vi "Decision2(SubVI).vi"(0 "L_ind0":i32, 1 "number of sample":i32, 2 "L_ind1":i32, 3 "Peak_ind0":dbl[](array[numeric]), 4 "index":i32, 5 "Peak_ind1":dbl[](array[numeric])) -> (6 "L_sum":i32, 7 "Bits":dbl[](array[numeric]), 8 "Position":dbl[](array[numeric]))   [LabVIEW 2017]
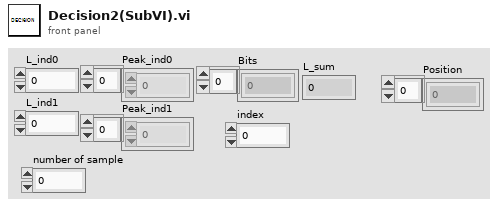
[diagram p1: front panel]
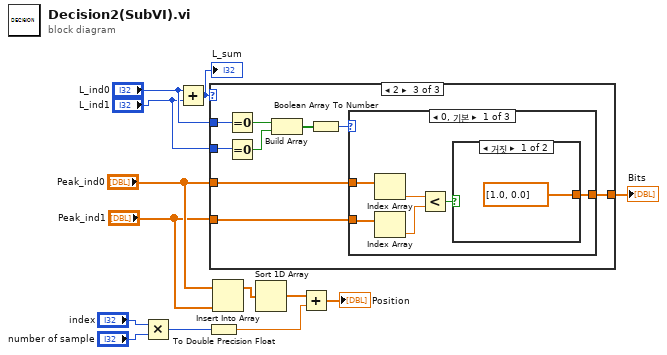
[diagram p0: block diagram]
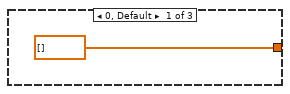
[diagram p2: hidden frame]
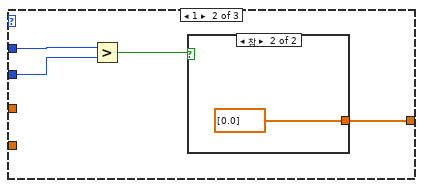
[diagram p3: hidden frame]
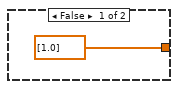
[diagram p4: hidden frame]
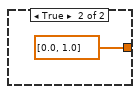
[diagram p5: hidden frame]
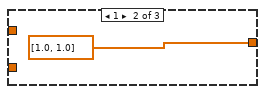
[diagram p6: hidden frame]
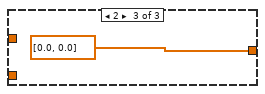
[diagram p7: hidden frame]
diagram:
  n1 = Multiply(x="index", y="number of sample") -> (x*y=w1:i32)
  n2 = Add(x="L_ind0", y="L_ind1") -> (x+y=w10:i32)
  "L_sum" <- w10
  n3 = To Double Precision Float(number=w1) -> (double precision float=w5:dbl)
  n4 = case shown="2" w10 {
    tunnel: [dbl[] [] w17 w23] -> w11
    tunnel: "L_ind0" -> [_ w16 w29]
    tunnel: "L_ind1" -> [_ w15 w28]
    tunnel: "Peak_ind0" -> [_ _ w22]
    tunnel: "Peak_ind1" -> [_ _ w21]
    frame 0, Default {
    }
    frame 1 {
      n5 = Greater?(x=w16, y=w15) -> (0:w18:bool)
      n6 = case shown="참" w18 {
        tunnel: [dbl[] [1.0] dbl[] [0.0]] -> w17
        frame False {
        }
        frame True {
        }
      }
    }
    frame 2 {
      n7 = Equal To 0?(x=w29) -> (x = 0?=w27:bool)
      n8 = Equal To 0?(x=w28) -> (x = 0?=w26:bool)
      n9 = Build Array(w27, w26) -> (w25:bool[])
      n10 = Boolean Array To Number(Boolean array=w25) -> (number=w24:u32)
      n11 = case shown="0, 기본" w24 {
        tunnel: [w30 dbl[] [1.0, 1.0] dbl[] [0.0, 0.0]] -> w23
        tunnel: w22 -> [w35 _ _]
        tunnel: w21 -> [w34 _ _]
        frame 0, Default {
          n12 = Index Array(array=w35) -> (element=w33:dbl)  [unwired: 1 in]
          n13 = Index Array(array=w34) -> (element=w32:dbl)  [unwired: 1 in]
          n14 = Less?(x=w33, y=w32) -> (x < y?=w31:bool)
          n15 = case shown="거짓" w31 {
            tunnel: [dbl[] [1.0, 0.0] dbl[] [0.0, 1.0]] -> w30
            frame False {
            }
            frame True {
            }
          }
        }
        frame 1 {
        }
        frame 2 {
        }
      }
    }
  }
  "Bits" <- w11
  n16 = Insert Into Array(array="Peak_ind0", new element="Peak_ind1") -> (w7:dbl[])  [unwired: 1 in]
  n17 = Sort 1D Array(array=w7) -> (sorted array=w6:dbl[])
  n18 = Add(x=w6, y=w5) -> (x+y=→"Position":dbl[])
